vi "String To Hex（6位）.vi"(11 "String":string) -> (0 "高低对调数据":string, 1 "高位":string, 2 "低位":string, 3 "Hex":string)   [LabVIEW 2017]
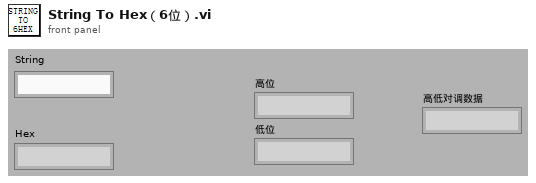
[diagram p1: front panel]
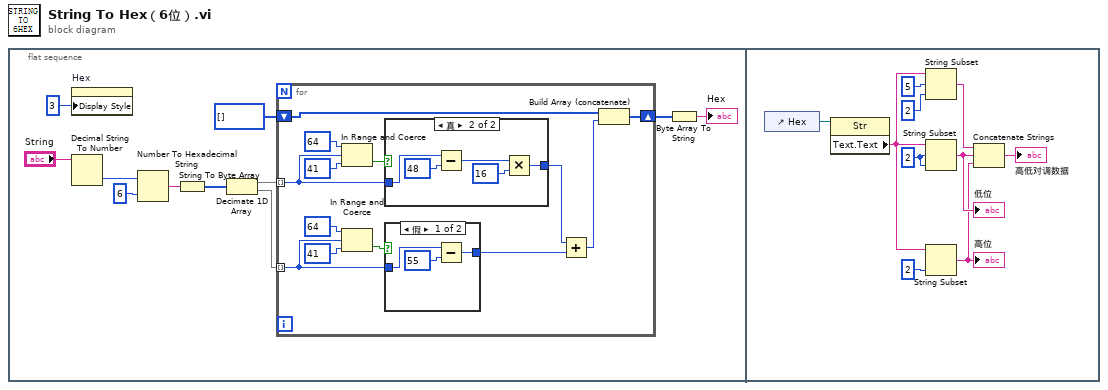
[diagram p0: block diagram]
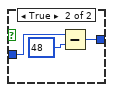
[diagram p2: hidden frame]
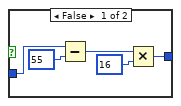
[diagram p3: hidden frame]
diagram:
  n1 = flat-sequence {
    frame #0 {
      n2 = property on="Hex" class="Str"("Display Style"=u32 3 ("显示样式")) -> ()  [unwired: 2 in, 2 out]
      n3 = Decimal String To Number(string="String") -> (number=w10:i32)  [unwired: 2 in, 1 out]
      n4 = Number To Hexadecimal String(1:i16 6 ("宽度(-)"), 2:w10) -> (0:w4:string)
      n5 = String To Byte Array(string=w4) -> (unsigned byte array=w7:u8[])
      n6 = Decimate 1D Array(w7) -> (w6:u8[], w5:u8[])
      n7 = for {
        shift-right: [w14] -> w2
        shift-left: u8[] [] -> [w16]
        tunnel: w6 -> [w13] mode=indexing
        tunnel: w5 -> [w12] mode=indexing
        n8 = In Range and Coerce(upper limit=u8 64 ("上限"), x=w13, lower limit=u8 41 ("下限")) -> (In Range?=w22:bool)  [unwired: 1 out]
        n9 = In Range and Coerce(upper limit=u8 64 ("上限"), x=w12, lower limit=u8 41 ("下限")) -> (In Range?=w19:bool)  [unwired: 1 out]
        n10 = case shown="真" w22 {
          tunnel: w13 -> [w32 w36]
          tunnel: [w31 w37] -> w18
          frame False {
            n11 = Subtract(x=w32, y=u8 55 ("上限")) -> (x-y=w34:u8)
            n12 = Multiply(x=w34, y=u8 16 ("上限")) -> (x*y=w31:u8)
          }
          frame True {
            n13 = Subtract(x=w36, y=u8 48 ("上限")) -> (x-y=w39:u8)
            n14 = Multiply(x=w39, y=u8 16 ("上限")) -> (x*y=w37:u8)
          }
        }
        n15 = case shown="假" w19 {
          tunnel: w12 -> [w25 w29]
          tunnel: [w26 w28] -> w17
          frame False {
            n16 = Subtract(x=w25, y=u8 55 ("上限")) -> (x-y=w26:u8)
          }
          frame True {
            n17 = Subtract(x=w29, y=u8 48 ("上限")) -> (x-y=w28:u8)
          }
        }
        n18 = Add(x=w18, y=w17) -> (x+y=w15:u8)
        n19 = Build Array (concatenate)(w16, w15) -> (w14:u8[])
      }
      n20 = Byte Array To String(unsigned byte array=w2) -> (string=→"Hex":string)
    }
    frame #1 {
      w48 = 2 ("长度（剩余）")
      n21 = control-ref of="Hex"() -> (w50:refnum<vi>)
      n22 = property class="Str"(reference=w50) -> ("Text.Text"=w43:string)  [unwired: 1 in, 2 out]
      n23 = String Subset(string=w43, offset (0)=5 ("偏移量(0)"), length (rest)=2 ("长度（剩余）")) -> (substring=w41:string)
      n24 = String Subset(string=w43, offset (0)=w48, length (rest)=w48) -> (substring=w47:string)
      "低位" <- w47
      n25 = String Subset(string=w43, length (rest)=2 ("长度（剩余）")) -> (substring=w44:string)  [unwired: 1 in]
      "高位" <- w44
      n26 = Concatenate Strings(w41, w47, w44) -> (→"高低对调数据":string)
    }
  }
